vi "Check Events.vi"(8 "error in (no error)":errorcluster, 11 "PluginGUI in":refnum<class "PluginGUI.lvclass">) -> (0 "error out":errorcluster, 3 "PluginGUI out":refnum<class "PluginGUI.lvclass">)   [LabVIEW 2020, in "VolatusGUI.lvlib" / "PluginGUI.lvclass"]
uses:
  PluginGUI.lvclass
  C:/dev/lv20CE/relink/lv-volatus/Volatus/Module/Module.lvclass
  PluginGUI.lvclass/PluginGUI.ctl
  OnValueChangeHandler/OnValueChangeHandler.lvclass
  Volatus/Module/Module.lvclass/Module.ctl
  OnMouseDown/OnMouseDown.lvclass
  Volatus/Module/Module.lvclass
  C:/dev/lv20CE/relink/lv-volatus/VolatusGUI/PluginGUI/PluginGUI.lvclass
  Volatus/VolatusAPI/VolatusAPI.lvclass
  Volatus/Volatus.lvlib
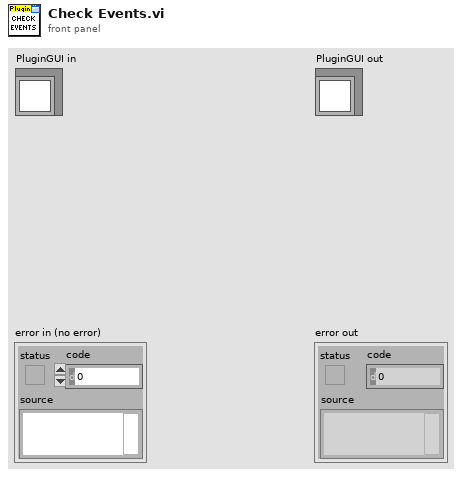
[diagram p1: front panel]
types:
  T1 = typedef "LVPoint32TypeDef.ctl" = cluster{"Horizontal":i32, "Vertical":i32}
  T2 = cluster{"Shift":bool, "Ctrl":bool, "Alt":bool, "Cmd":bool, "Opt":bool}
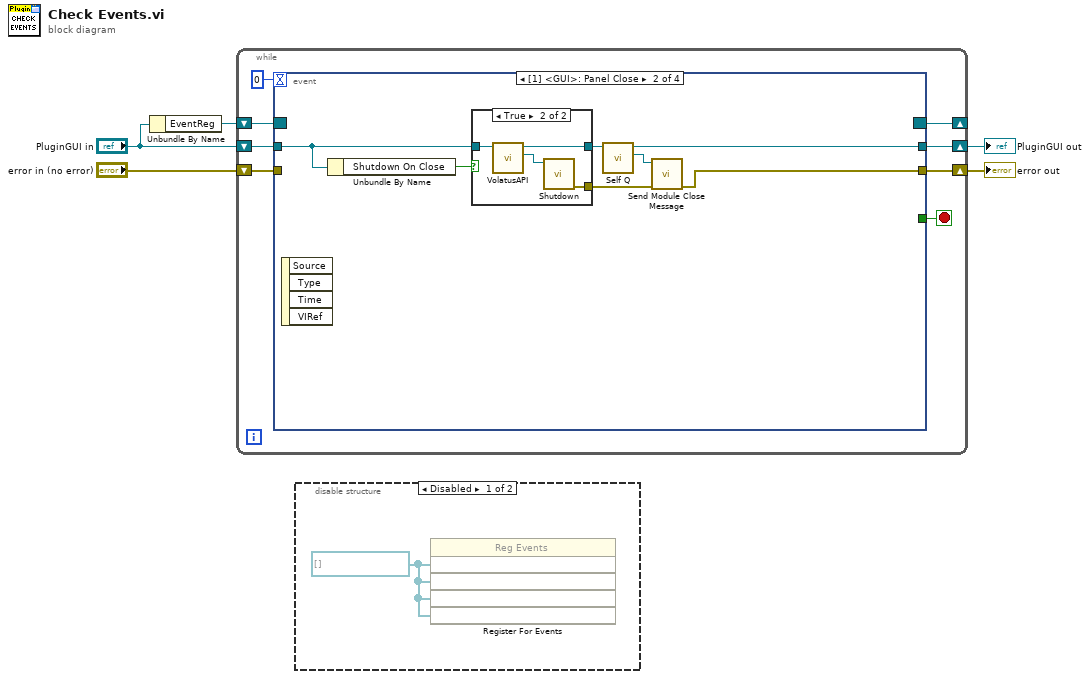
[diagram p0: block diagram]
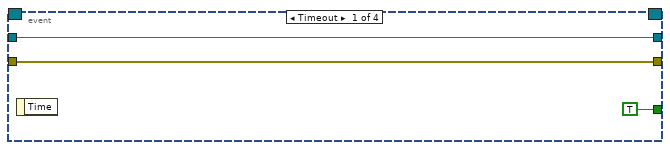
[diagram p3: hidden frame]
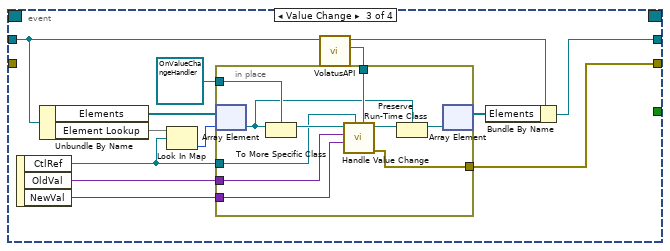
[diagram p5: hidden frame]
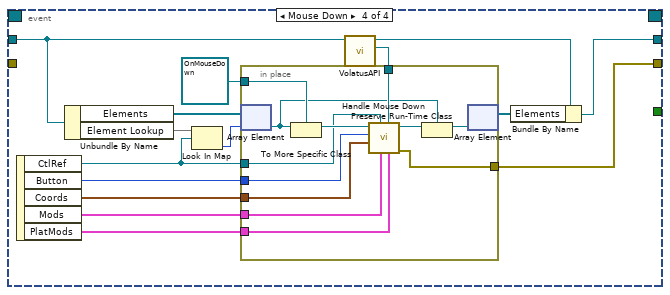
[diagram p6: hidden frame]
diagram:
  n1 = Unbundle By Name("PluginGUI in") -> ("EventReg"=w4:refnum<event-registration>)
  n2 = while {
    shift-right: [w8] -> w2
    shift-left: "PluginGUI in" -> [w11]
    shift-right: [w12] -> _
    shift-left: w4 -> [w13]
    shift-right: [w7] -> w1
    shift-left: "error in (no error)" -> [w10]
    stop <- w6 stop-if-true
    n3 = event shown="[1] <GUI>: Panel Close" {
      selector: w13 -> [_ _ _ _]
      dyn-events: [_ _ _ _] -> w12
      timeout: 0 -> [_ _ _ _]
      tunnel: w11 -> [w16 w22 w36 w52]
      tunnel: w10 -> [w15 _ _ _]
      tunnel: [w16 w20 w30 w58] -> w8
      tunnel: [w15 w17 w31 w59] -> w7
      tunnel: [TRUE _ _ _] -> w6
      event Timeout {
        n4 = event-data() -> ()  [unwired: 1 in, 1 out]
      }
      event Panel Close {
        n5 = event-data() -> ()  [unwired: 1 in, 4 out]
        n6 = Unbundle By Name(w22) -> ("Shutdown On Close"=w23:bool)
        n7 = case shown="True" w23 {
          tunnel: w22 -> [w24 w28]
          tunnel: [w24 w26] -> w21
          tunnel: [_ w25] -> w18
          frame False {
          }
          frame True {
            n8 = call "VolatusAPI.vi"("Module in"=w28) -> ("VolatusAPI"=w27:refnum<class "VolatusAPI.lvclass">, "Module out"=w26:refnum<class "PluginGUI.lvclass">)  [unwired: 9 in]
            n9 = call "Shutdown.vi"("VolatusAPI in"=w27) -> ("error out"=w25:errorcluster)  [unwired: 9 in, 1 out]
          }
        }
        n10 = call "Self Q.vi"("Module in"=w21) -> ("Self Q"=w19:refnum<class "MessageQ.lvclass">, "Module out"=w20:refnum<class "PluginGUI.lvclass">)  [unwired: 9 in]
        n11 = call "Send Module Close Message.vi"("error in (no error)"=w18, "MessageQ"=w19) -> ("error out"=w17:errorcluster)  [unwired: 9 in]
      }
      event Value Change {
        n12 = event-data() -> ("CtlRef"=w37:refnum<vi>, "OldVal"=w33:variant, "NewVal"=w32:variant)  [unwired: 1 in]
        n13 = Unbundle By Name(w36) -> ("Elements"=w40:refnum<class "GUI Element.lvclass">[], "Element Lookup"=w41:map{refnum<vi>, i32})
        n14 = Look In Map(map=w41, key=w37) -> (value=w39:i32)  [unwired: 1 in, 1 out]
        n15 = call "VolatusAPI.vi"("Module in"=w36) -> ("VolatusAPI"=w35:refnum<class "VolatusAPI.lvclass">, "Module out"=w34:refnum<class "PluginGUI.lvclass">)  [unwired: 9 in]
        n16 = in-place {
          in-place-border: refnum<class "OnValueChangeHandler.lvclass"> refnum ("OnValueChangeHandler in") -> [w50]
          in-place-border: w37 -> [w49]
          in-place-border: w35 -> [w48]
          in-place-border: w33 -> [w47]
          in-place-border: w32 -> [w46]
          in-place-border: [w42] -> w31
          n17 = in-place-array #1(w40, w39) -> (w43:refnum<class "GUI Element.lvclass">)
          n18 = To More Specific Class(target class=w50, reference=w43) -> (specific class reference=w51:refnum<class "OnValueChangeHandler.lvclass">)  [unwired: 1 in, 1 out]
          n19 = call-dynamic "Handle Value Change.vi"("VolatusAPI"=w48, "CtlRef"=w49, "NewVal"=w46, "OldVal"=w47, "OnValueChangeHandler in"=w51) -> ("error out"=w42:errorcluster, "OnValueChangeHandler out"=w45:refnum<class "OnValueChangeHandler.lvclass">)  [unwired: 5 in]
          n20 = Preserve Run-Time Class(object in=w45, 2:w43) -> (object out=w44:refnum<class "GUI Element.lvclass">)  [unwired: 1 in, 1 out]
          n21 = in-place-array #1(w44) -> (w29:refnum<class "GUI Element.lvclass">[])  [unwired: 1 out]
        }
        n22 = Bundle By Name(cluster=w34, "Elements"=w29) -> (w30:refnum<class "PluginGUI.lvclass">)
      }
      event Mouse Down {
        n23 = event-data() -> ("CtlRef"=w57:refnum<vi>, "Button"=w56:u16, "Coords"=w55:T1, "Mods"=w54:cluster{"Double Click":bool, "Menu Key":bool}, "PlatMods"=w53:T2)  [unwired: 1 in]
        n24 = Unbundle By Name(w52) -> ("Elements"=w65:refnum<class "GUI Element.lvclass">[], "Element Lookup"=w66:map{refnum<vi>, i32})
        n25 = Look In Map(map=w66, key=w57) -> (value=w64:i32)  [unwired: 1 in, 1 out]
        n26 = call "VolatusAPI.vi"("Module in"=w52) -> ("VolatusAPI"=w62:refnum<class "VolatusAPI.lvclass">, "Module out"=w61:refnum<class "PluginGUI.lvclass">)  [unwired: 9 in]
        n27 = in-place {
          in-place-border: refnum<class "OnMouseDown.lvclass"> refnum ("OnValueChangeHandler in") -> [w77]
          in-place-border: w57 -> [w76]
          in-place-border: w62 -> [w75]
          in-place-border: [w71] -> w59
          in-place-border: w56 -> [w70]
          in-place-border: w55 -> [w69]
          in-place-border: w54 -> [w68]
          in-place-border: w53 -> [w67]
          n28 = in-place-array #2(w65, w64) -> (w72:refnum<class "GUI Element.lvclass">)
          n29 = To More Specific Class(target class=w77, reference=w72) -> (specific class reference=w78:refnum<class "OnMouseDown.lvclass">)  [unwired: 1 in, 1 out]
          n30 = call-dynamic "Handle Mouse Down.vi"("PlatMods"=w67, "VolatusAPI"=w75, "Mods"=w68, "CtlRef"=w76, "Coords"=w69, "Button"=w70, "OnMouseDown in"=w78) -> ("error out"=w71:errorcluster, "OnMouseDown out"=w74:refnum<class "OnMouseDown.lvclass">)  [unwired: 3 in]
          n31 = Preserve Run-Time Class(object in=w74, 2:w72) -> (object out=w73:refnum<class "GUI Element.lvclass">)  [unwired: 1 in, 1 out]
          n32 = in-place-array #2(w73) -> (w60:refnum<class "GUI Element.lvclass">[])  [unwired: 1 out]
        }
        n33 = Bundle By Name(cluster=w61, "Elements"=w60) -> (w58:refnum<class "PluginGUI.lvclass">)
      }
    }
  }
  "error out" <- w1
  "PluginGUI out" <- w2
  n34 = disable-structure shown="Disabled" {
    frame Disabled {
      w79 = refnum<vi>[] []
      n35 = register-events(w79, w79, w79, w79) -> ()  [unwired: 2 in, 2 out]
    }
    frame Enabled {
    }
  }
